vi "integrator.vi"(11 "Signal":i64[](array[numeric])) -> (3 "Result":dynamicdata(waveform))   [LabVIEW 2016]
uses:
  <vilib>/Analysis/baseanly.llb/Mean (DBL).vi
  <vilib>/Analysis/NI_AALBase.lvlib
panel:
  # "De-means the signal\nand integrates it"
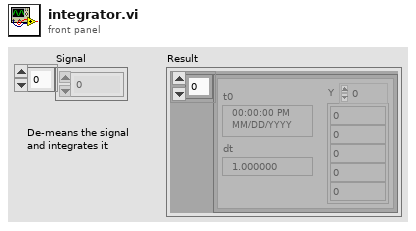
[diagram p1: front panel]
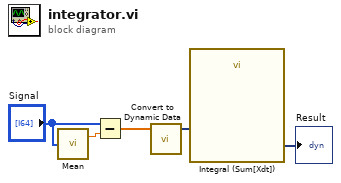
[diagram p0: block diagram]
diagram:
  n1 = call-poly <vilib>:"Mean.vi"("X"="Signal") -> ("mean"=w1:dbl)  [unwired: 1 out]
  n2 = Subtract(x="Signal", y=w1) -> (x-y=w2:dbl[])
  n3 = call "Convert to Dynamic Data"("Array"=w2) -> ("Dynamic Data Type"=w3:dynamicdata)  [unwired: 3 in]
  n4 = call "Integral (Sum[Xdt])"("Signals"=w3) -> ("Result"=→"Result":dynamicdata)  [unwired: 5 in, 1 out]
